vi "MultiChannelFeedbackCooling_aod_feedback(Host).vi"(5 "RIO Device":T1="RIO0") -> ()   [LabVIEW 2014]
doc: "This VI will will initialize the FPGA VI and then continually read and convert single point values from 4 channels of an analog input module."
uses:
  <vilib>/userdefined/High Color/nirio_resource_hc.ctl
  <vilib>/rvi/Analysis/host/Butterworth/config/Butterworth Filter Order.ctl
  <vilib>/rvi/Analysis/host/Butterworth/config/Butterworth Filter Type.ctl
  <vilib>/FPGAPlugInAG/PXI-7854R/niLvFpga_Open_PXI-7854R.vi
  <vilib>/FPGAPlugInAG/PXI-7854R/niLvFpga_Run_PXI-7854R.vi
  <vilib>/rvi/Analysis/host/Butterworth/config/BwScaledCoefficients.vi
  <vilib>/Utility/error.llb/Error Cluster From Error Code.vi
  <vilib>/rvi/errors/niLvFpgaAdjustHostInterfaceError.vi
  <vilib>/Utility/file.llb/Read From Spreadsheet File (I64).vi
  <vilib>/FPGAPlugInAG/PXI-7854R/niLvFpga_Close_PXI-7854R.vi
  <vilib>/rvi/interface/nirviOpenFPGA/nirviOpenFPGA.xnode
  FPGA Bitfiles/MultiChannelFeed_FPGATarget_MultiChannelfFee_WCKCUTTT7ag.lvbitx
  MultiChannelfFeedbackCooling (FPGA).vi
  <vilib>/rvi/interface/nirviMethod/nirviMethod.xnode
  <vilib>/rvi/Analysis/host/Butterworth/XNode/ButterworthCoefficients.xnode
  <vilib>/rvi/interface/nirviReadWriteControl/nirviReadWriteControl.xnode
  <vilib>/rvi/interface/nirviCloseFPGA/nirviCloseFPGA.xnode
  NiFpgaLv.dll
  <vilib>/rvi/Analysis/host/Public/NI_FpgaMspHost.lvlib
panel:
  out "tot_fb_img":i16(graph)
  out "fb_img":i16(graph)
  out "AI_img":i16(graph)=3016
  in  "pg_img":fxp<+/-,24,12>
  in  "dg_img":fxp<+/-,24,12>
  in  "ig_img":fxp<+/-,24,6>
  in  "setpt_img":i16=3000
  in  "Upper lim_img":fxp<+/-,16,16>=1000.0
  in  "Lower lim_img":fxp<+/-,16,16>=-1000.0
  in  "lp freq_img":dbl=5000.0
  in  "hp freq_img":dbl=5000.0
  in  "output offset_img":i16
  in  "End value arb (ch1)":fxp<+/-,32,16>
  in  "Step arb (ch1)":fxp<+/-,32,16>=0.0005035400390625
  in  "Arb gain (ch2)":fxp<+/-,24,12>
  in  "z arb scale":fxp<+/-,33,17>
  in  "ramp arb drive":bool
  in  "End value arb (ch0)":fxp<+/-,32,16>
  in  "Step arb (ch0)":fxp<+/-,32,16>=0.0005035400390625
  in  "Delay Time (s) arb":dbl=0.001 caption="Delay Time (s)"
  in  "Buffer file path":path=path "C:/GitHub/opt_lev/labview/fpga/gauss_cdf.txt"
  in  "Write data to buffers":bool
  in  "Arb steps per cycle":u16=1
  in  "Arb gain (ch1)":fxp<+/-,24,12>
  in  "Arb gain (ch0)":fxp<+/-,24,12>
  in  "power setpt":i16=7000
  in  "Upper lim pow":fxp<+/-,16,16>=10000.0
  in  "Lower lim pow":fxp<+/-,16,16>=-10000.0
  in  "hp freq pow":dbl=5000.0
  in  "lp freq pow":dbl=5000.0
  in  "Use_PID2_power":bool=TRUE
  in  "hp freq 1":dbl=1100.0
  in  "hp freq 0":dbl=1100.0
  in  "lp freq 0":dbl=1100.0
  in  "DC offset 0":i16
  in  "Lower lim 0":fxp<+/-,16,16>=-3600.0
  in  "Upper lim 0":fxp<+/-,16,16>=3600.0
  in  "Dg 0":fxp<+/-,24,12>
  in  "Bead setpt 0":i16
  in  "change pars":bool
  in  "hp freq 2":dbl=1100.0
  in  "lp freq 1":dbl=1100.0
  in  "lp freq 2":dbl=1100.0
  in  "ramp power":bool
  in  "End value power":i16=1600
  in  "Step power":i16=5
  in  "Delay Time (s) power":dbl=0.01 caption="Delay Time (s)"
  in  "Count(usec)":u32=10
  in  "?":u16(ring)=2 items=["Both", "AOD", "Bead"]
  in  "?":u16(ring)=2 items=["Both", "AOD", "Bead"]
  in  "?":u16(ring) items=["Both", "AOD", "Bead"]
  in  "?":u16(ring)=2 items=["Both", "AOD", "Bead"]
  in  "?":u16(ring)=1 items=["Both", "AOD", "Bead"]
  in  "?":u16(ring)=2 items=["Both", "AOD", "Bead"]
  in  "Pg d2":fxp<+/-,24,12>=-6.0
  in  "Ig d2":fxp<+/-,24,6>=-0.7999992370605469
  in  "Dg d2":fxp<+/-,24,12>
  in  "Ig 2":fxp<+/-,24,6>
  in  "DC offset 2":i16=7000
  in  "Lower lim 2":fxp<+/-,16,16>=-2000.0
  in  "Upper lim 2":fxp<+/-,16,16>=2000.0
  in  "Dg 2":fxp<+/-,24,12>
  in  "Pg 2":fxp<+/-,24,12>
  in  "Bead setpt 2":i16=1000
  in  "change pars 2":bool
  in  "change pars 1":bool
  in  "DC offset 1":i16
  in  "Lower lim 1":fxp<+/-,16,16>=-32768.0
  in  "Upper lim 1":fxp<+/-,16,16>=32767.0
  in  "Dg 1":fxp<+/-,24,12>
  in  "Bead setpt 1":i16
  out "Tot feedback + DC, Ch2":i16(graph)=3860
  out "Individual feedback, Ch2":cluster{"fb_0":i16, "fb_d0":i16}(graph)
  out "AI1 2":cluster{"AI2":i16, "AI5":i16}(graph)={"AI2"=2178, "AI5"=2178}
  out "Tot feedback + DC, Ch1":i16(graph)
  out "Individual feedback, Ch1":cluster{"fb_0":i16, "fb_d0":i16}(graph)
  out "AI1":cluster{"AI1":i16, "AI4":i16}(graph)={"AI1"=-1988, "AI4"=-1988}
  out "Tot feedback + DC, Ch0":i16(graph)
  out "Individual feedback, Ch0":cluster{"fb_0":i16, "fb_d0":i16}(graph)
  out "AI0":cluster{"AI0":i16, "AI3":i16}(graph)={"AI0"=-128, "AI3"=-128}
  in  "stop":bool
  # "FPGA feedback GUI"
  # "Bead arbitrary drive:"
  # "PID controls, X (ch 0):"
  # "PID controls, Y (ch 1):"
  # "Bead feedback:"
  # "Bead feedback:"
  # "PID controls, Z (ch 2):"
  # "Bead feedback:"
  # "AOD feeback:"
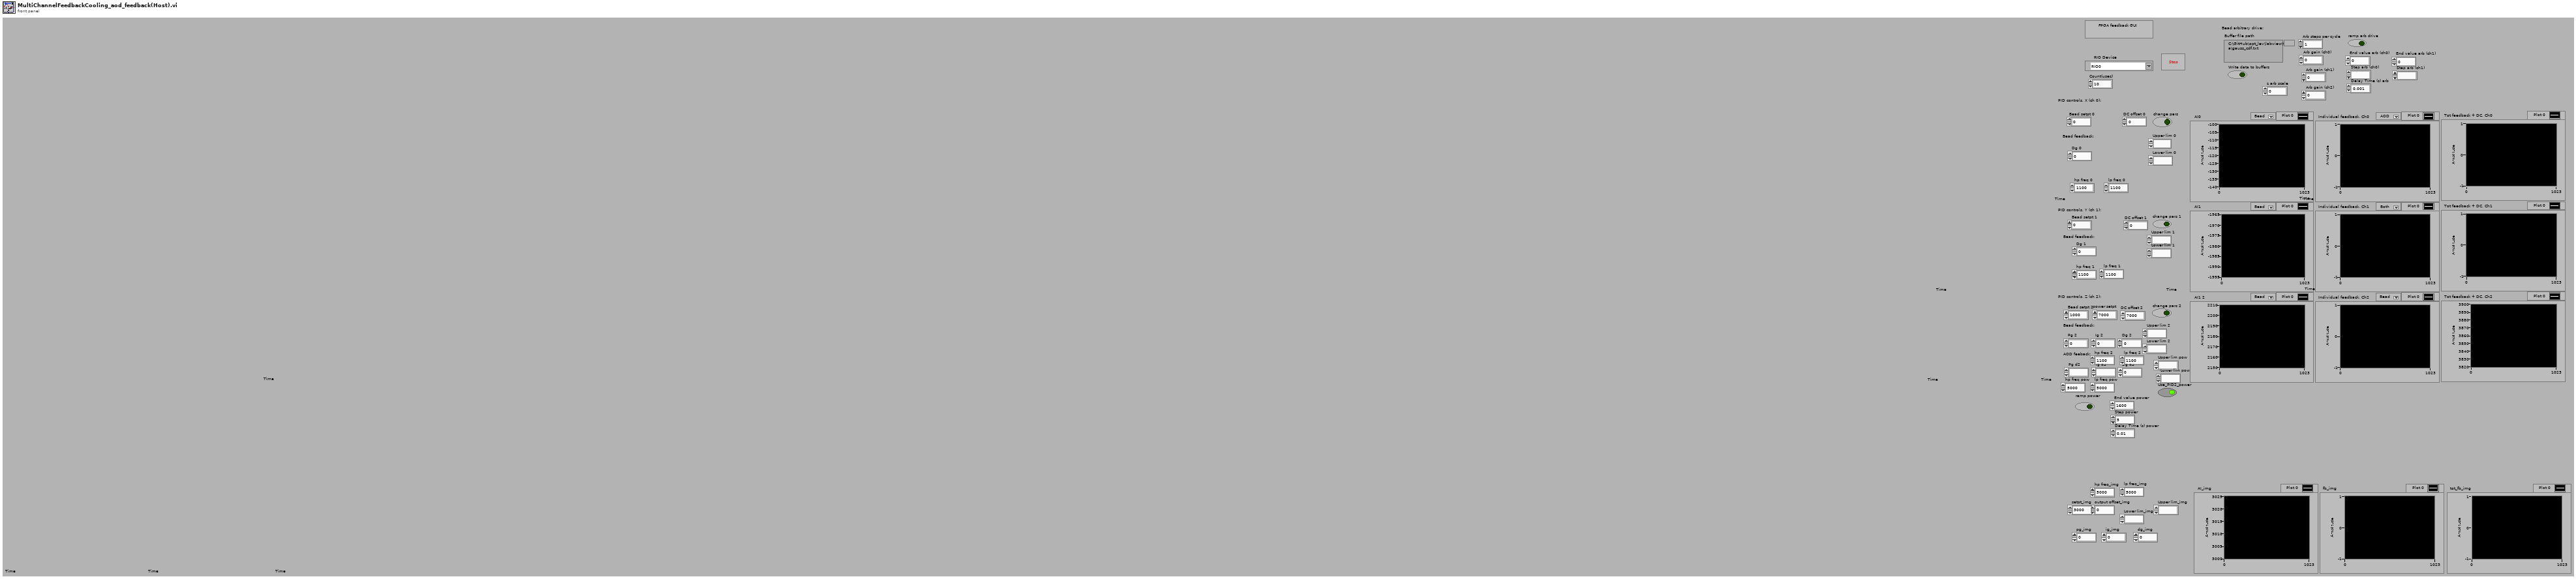
[diagram p1: front panel]
types:
  T1 = typedef "nirio_resource_hc.ctl" = tag
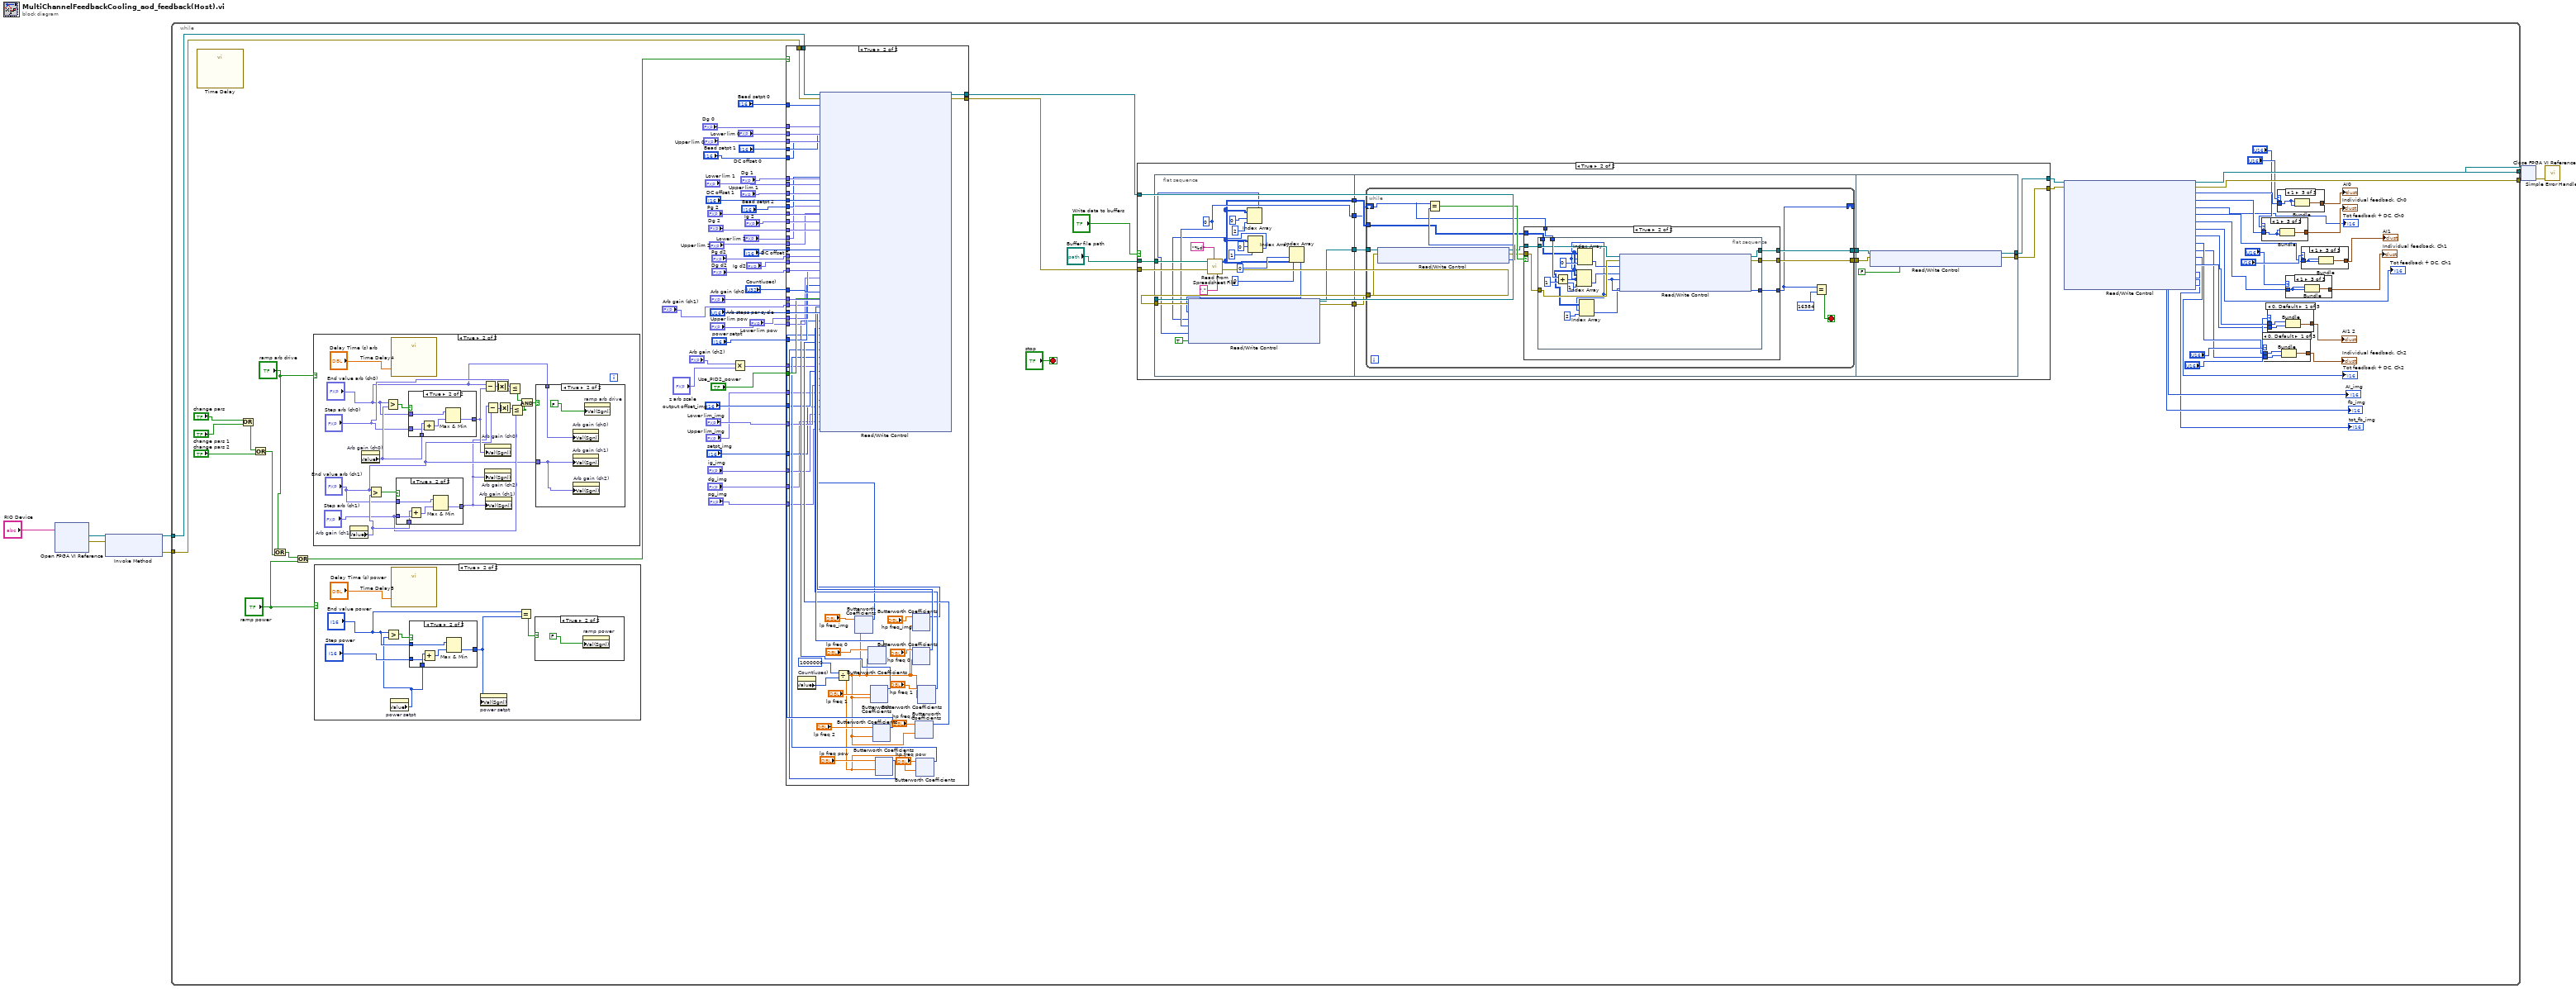
[diagram p0: block diagram]
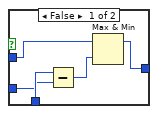
[diagram p4: hidden frame]
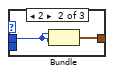
[diagram p5: hidden frame]
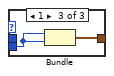
[diagram p6: hidden frame]
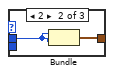
[diagram p7: hidden frame]
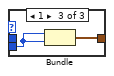
[diagram p8: hidden frame]
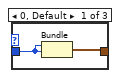
[diagram p9: hidden frame]
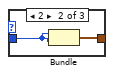
[diagram p10: hidden frame]
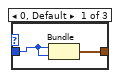
[diagram p11: hidden frame]
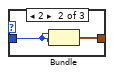
[diagram p12: hidden frame]
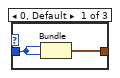
[diagram p13: hidden frame]
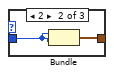
[diagram p14: hidden frame]
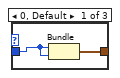
[diagram p15: hidden frame]
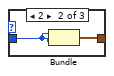
[diagram p16: hidden frame]
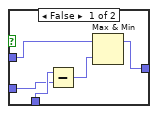
[diagram p18: hidden frame]
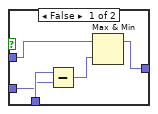
[diagram p20: hidden frame]
diagram:
  n1 = xnode "Open FPGA VI Reference"("resource name"="RIO Device") -> ("FPGA VI Reference Out"=w3:refnum<k20>, "error out"=w2:errorcluster)  [unwired: 1 in]
  n2 = xnode "Invoke Method"("FPGA VI Reference In"=w3, "error in"=w2) -> ("FPGA VI Reference Out"=w5:refnum<k20>, "error out"=w4:errorcluster)  [unwired: 1 in]
  n3 = while {
    tunnel: [w92] -> w8
    tunnel: w5 -> [w84]
    tunnel: w4 -> [w83]
    tunnel: [w91] -> w1
    stop <- "stop" stop-if-true
    n4 = call "Time Delay"() -> ()  [unwired: 11 in, 1 out]
    n5 = Or(x="change pars", y="change pars 1") -> (x .or. y?=w57:bool)
    n6 = Or(x=w57, y="change pars 2") -> (x .or. y?=w23:bool)
    n7 = Or(x="ramp arb drive", y=w23) -> (x .or. y?=w30:bool)
    n8 = Or(x=w30, y="ramp power") -> (x .or. y?=w31:bool)
    n9 = case shown="True" "ramp arb drive" {
      frame False {
      }
      frame True {
        n10 = property on="Arb gain (ch1)" class="DigNum (strict)"() -> ("Value"=w162:fxp<+/-,24,12>)  [unwired: 2 in, 2 out]
        n11 = property on="Arb gain (ch0)" class="DigNum (strict)"() -> ("Value"=w165:fxp<+/-,24,12>)  [unwired: 2 in, 2 out]
        n12 = Greater?(x="End value arb (ch1)", y=w162) -> (0:w163:bool)
        n13 = Greater?(x="End value arb (ch0)", y=w165) -> (0:w166:bool)
        n14 = call "Time Delay4"("Delay Time (s)"="Delay Time (s) arb") -> ()  [unwired: 10 in, 1 out]
        n15 = case shown="True" w163 {
          tunnel: "End value arb (ch1)" -> [w168 w174]
          tunnel: w162 -> [w171 w172]
          tunnel: "Step arb (ch1)" -> [w170 w176]
          tunnel: [w167 w173] -> w149
          frame False {
            n16 = Subtract(x=w171, y=w170) -> (x-y=w169:fxp<+/-,33,17>)
            n17 = Max & Min(x=w168, y=w169) -> (max(x,y)=w167:fxp<+/-,33,17>)  [unwired: 1 out]
          }
          frame True {
            n18 = Add(x=w172, y=w176) -> (x+y=w175:fxp<+/-,33,17>)
            n19 = Max & Min(x=w174, y=w175) -> (min(x,y)=w173:fxp<+/-,33,17>)  [unwired: 1 out]
          }
        }
        n20 = case shown="True" w166 {
          tunnel: "End value arb (ch0)" -> [w181 w186]
          tunnel: w165 -> [w184 w189]
          tunnel: "Step arb (ch0)" -> [w183 w188]
          tunnel: [w180 w185] -> w161
          frame False {
            n21 = Subtract(x=w184, y=w183) -> (x-y=w182:fxp<+/-,33,17>)
            n22 = Max & Min(x=w181, y=w182) -> (max(x,y)=w180:fxp<+/-,33,17>)  [unwired: 1 out]
          }
          frame True {
            n23 = Add(x=w189, y=w188) -> (x+y=w187:fxp<+/-,33,17>)
            n24 = Max & Min(x=w186, y=w187) -> (min(x,y)=w185:fxp<+/-,33,17>)  [unwired: 1 out]
          }
        }
        n25 = Subtract(x="End value arb (ch0)", y=w161) -> (x-y=w160:fxp<+/-,34,18>)
        n26 = property on="Arb gain (ch0)" class="DigNum (strict)"("Val(Sgnl)"=w161) -> ()  [unwired: 2 in, 2 out]
        n27 = property on="Arb gain (ch2)" class="DigNum (strict)"("Val(Sgnl)"=w149) -> ()  [unwired: 2 in, 2 out]
        n28 = Subtract(x=w149, y="End value arb (ch1)") -> (x-y=w157:fxp<+/-,34,18>)
        n29 = property on="Arb gain (ch1)" class="DigNum (strict)"("Val(Sgnl)"=w149) -> ()  [unwired: 2 in, 2 out]
        n30 = Absolute Value(x=w160) -> (abs(x)=w159:fxp<+,33,17>)
        n31 = Absolute Value(x=w157) -> (abs(x)=w156:fxp<+,33,17>)
        n32 = Less Or Equal?(x=w159, y="Step arb (ch0)") -> (x <= y?=w153:bool)
        n33 = Less Or Equal?(x=w156, y="Step arb (ch1)") -> (x <= y?=w152:bool)
        n34 = And(x=w153, y=w152) -> (x .and. y?=w154:bool)
        n35 = case shown="True" w154 {
          tunnel: "End value arb (ch0)" -> [_ w178]
          tunnel: "End value arb (ch1)" -> [_ w177]
          frame False {
          }
          frame True {
            n36 = property on="Arb gain (ch0)" class="DigNum (strict)"("Val(Sgnl)"=w178) -> ()  [unwired: 2 in, 2 out]
            n37 = property on="Arb gain (ch1)" class="DigNum (strict)"("Val(Sgnl)"=w177) -> ()  [unwired: 2 in, 2 out]
            n38 = property on="Arb gain (ch2)" class="DigNum (strict)"("Val(Sgnl)"=w177) -> ()  [unwired: 2 in, 2 out]
            n39 = property on="ramp arb drive" class="Bool (strict)"("Val(Sgnl)"=FALSE) -> ()  [unwired: 2 in, 2 out]
          }
        }
      }
    }
    n40 = case shown="True" "ramp power" {
      frame False {
      }
      frame True {
        n41 = property on="power setpt" class="DigNum (strict)"() -> ("Value"=w94:i16)  [unwired: 2 in, 2 out]
        n42 = Greater?(x="End value power", y=w94) -> (0:w99:bool)
        n43 = call "Time Delay5"("Delay Time (s)"="Delay Time (s) power") -> ()  [unwired: 10 in, 1 out]
        n44 = case shown="True" w99 {
          tunnel: "End value power" -> [w102 w107]
          tunnel: w94 -> [w105 w110]
          tunnel: "Step power" -> [w104 w109]
          tunnel: [w101 w106] -> w93
          frame False {
            n45 = Subtract(x=w105, y=w104) -> (x-y=w103:i16)
            n46 = Max & Min(x=w102, y=w103) -> (max(x,y)=w101:i16)  [unwired: 1 out]
          }
          frame True {
            n47 = Add(x=w110, y=w109) -> (x+y=w108:i16)
            n48 = Max & Min(x=w107, y=w108) -> (min(x,y)=w106:i16)  [unwired: 1 out]
          }
        }
        n49 = property on="power setpt" class="DigNum (strict)"("Val(Sgnl)"=w93) -> ()  [unwired: 2 in, 2 out]
        n50 = Equal?(x="End value power", y=w93) -> (x = y?=w98:bool)
        n51 = case shown="True" w98 {
          frame False {
          }
          frame True {
            n52 = property on="ramp power" class="Bool (strict)"("Val(Sgnl)"=FALSE) -> ()  [unwired: 2 in, 2 out]
          }
        }
      }
    }
    n53 = Multiply(x="Arb gain (ch2)", y="z arb scale") -> (x*y=w20:fxp<+/-,56,28>)
    n54 = case shown="True" w31 {
      tunnel: w83 -> [w271 w326]
      tunnel: [w271 w334] -> w79
      tunnel: [w270 w333] -> w80
      tunnel: "Bead setpt 0" -> [_ w332]
      tunnel: "Dg 0" -> [_ w331]
      tunnel: "Upper lim 0" -> [_ w329]
      tunnel: "Lower lim 0" -> [_ w330]
      tunnel: "DC offset 0" -> [_ w328]
      tunnel: w84 -> [w270 w327]
      tunnel: "Bead setpt 1" -> [_ w325]
      tunnel: "Dg 1" -> [_ w324]
      tunnel: "Lower lim 1" -> [_ w323]
      tunnel: "Upper lim 1" -> [_ w322]
      tunnel: "DC offset 1" -> [_ w321]
      tunnel: "Bead setpt 2" -> [_ w320]
      tunnel: "Pg 2" -> [_ w319]
      tunnel: "Ig 2" -> [_ w318]
      tunnel: "Dg 2" -> [_ w317]
      tunnel: "Lower lim 2" -> [_ w316]
      tunnel: "Upper lim 2" -> [_ w315]
      tunnel: "DC offset 2" -> [_ w314]
      tunnel: "Pg d2" -> [_ w313]
      tunnel: "Ig d2" -> [_ w312]
      tunnel: "Dg d2" -> [_ w311]
      tunnel: "Arb gain (ch0)" -> [_ w310]
      tunnel: "Arb gain (ch1)" -> [_ w296]
      tunnel: "Arb steps per cycle" -> [_ w309]
      tunnel: "Count(usec)" -> [_ w308]
      tunnel: "Use_PID2_power" -> [_ w299]
      tunnel: "Lower lim pow" -> [_ w295]
      tunnel: "Upper lim pow" -> [_ w294]
      tunnel: "power setpt" -> [_ w293]
      tunnel: w20 -> [_ w284]
      tunnel: "output offset_img" -> [_ w283]
      tunnel: "Lower lim_img" -> [_ w278]
      tunnel: "Upper lim_img" -> [_ w277]
      tunnel: "setpt_img" -> [_ w275]
      tunnel: "ig_img" -> [_ w274]
      tunnel: "dg_img" -> [_ w273]
      tunnel: "pg_img" -> [_ w272]
      frame False {
      }
      frame True {
        n55 = property on="Count(usec)" class="DigNum (strict)"() -> ("Value"=w304:u32)  [unwired: 2 in, 2 out]
        n56 = Divide(x=u32 1000000, y=w304) -> (x/y=w281:dbl)
        n57 = xnode "Butterworth Coefficients"("cutoff frequency (Hz)"="lp freq_img", "sample rate (S/s)"=w281) -> ("scaled coefficients"=w276:i32[])  [unwired: 1 in, 1 out]
        n58 = xnode "Butterworth Coefficients"("cutoff frequency (Hz)"="lp freq 0", "sample rate (S/s)"=w281) -> ("scaled coefficients"=w292:i32[])  [unwired: 1 in, 1 out]
        n59 = xnode "Butterworth Coefficients"("cutoff frequency (Hz)"="lp freq 1", "sample rate (S/s)"=w281) -> ("scaled coefficients"=w290:i32[])  [unwired: 1 in, 1 out]
        n60 = xnode "Butterworth Coefficients"("cutoff frequency (Hz)"="lp freq 2", "sample rate (S/s)"=w281) -> ("scaled coefficients"=w288:i32[])  [unwired: 1 in, 1 out]
        n61 = xnode "Butterworth Coefficients"("cutoff frequency (Hz)"="lp freq pow", "sample rate (S/s)"=w281) -> ("scaled coefficients"=w286:i32[])  [unwired: 1 in, 1 out]
        n62 = xnode "Butterworth Coefficients"("cutoff frequency (Hz)"="hp freq_img", "sample rate (S/s)"=w281) -> ("scaled coefficients"=w279:i32[])  [unwired: 1 in, 1 out]
        n63 = xnode "Butterworth Coefficients"("cutoff frequency (Hz)"="hp freq 0", "sample rate (S/s)"=w281) -> ("scaled coefficients"=w291:i32[])  [unwired: 1 in, 1 out]
        n64 = xnode "Butterworth Coefficients"("cutoff frequency (Hz)"="hp freq 2", "sample rate (S/s)"=w281) -> ("scaled coefficients"=w287:i32[])  [unwired: 1 in, 1 out]
        n65 = xnode "Butterworth Coefficients"("cutoff frequency (Hz)"="hp freq pow", "sample rate (S/s)"=w281) -> ("scaled coefficients"=w285:i32[])  [unwired: 1 in, 1 out]
        n66 = xnode "Butterworth Coefficients"("cutoff frequency (Hz)"="hp freq 1", "sample rate (S/s)"=w281) -> ("scaled coefficients"=w289:i32[])  [unwired: 1 in, 1 out]
        n67 = xnode "Read/Write Control"("FPGA VI Reference In"=w327, "error in"=w326, "Dc Pos 0"=w332, "dg 0"=w331, "Lower lim 0"=w330, "Upper lim 0"=w329, "output offset 0"=w328, "Dc Pos 1"=w325, "dg 1"=w324, "Lower lim 1"=w323, "Upper lim 1"=w322, "output offset 1"=w321, "Dc Pos 2"=w320, "pg 2"=w319, "ig 3"=w318, "dg 2"=w317, "Lower lim 2"=w316, "Upper lim 2"=w315, "output offset 2"=w314, "pg d0 3"=w313, "ig d03"=w312, "dg d0 3"=w311, "Arb gain (ch0)"=w310, "Arb gain (ch1)"=w296, "Arb steps per cycle"=w309, "Lower lim 4"=w295, "Upper lim d0 3"=w294, "Dc Pos d2"=w293, "Count(uSec)"=w308, "Use_PID2_X 2"=w299, "lp coeff 0"=w292, "hp coeff 0"=w291, "lp coeff 1"=w290, "hp coeff 1"=w289, "lp coeff 2"=w288, "hp coeff 2"=w287, "lp coeff d2"=w286, "hp coeff d2"=w285, "Arb gain (ch2)"=w284, "output offset_img"=w283, "hp coeff_img"=w279, "Lower lim_img"=w278, "Upper lim_img"=w277, "lp coeff_img"=w276, "setpt_img"=w275, "ig_img"=w274, "dg_img"=w273, "pg_img"=w272) -> ("FPGA VI Reference Out"=w333:refnum<k20>, "error out"=w334:errorcluster)
      }
    }
    n68 = case shown="True" "Write data to buffers" {
      tunnel: "Buffer file path" -> [_ w202]
      tunnel: w80 -> [w191 w201]
      tunnel: w79 -> [w190 w200]
      tunnel: [w191 w193] -> w78
      tunnel: [w190 w192] -> w77
      frame False {
      }
      frame True {
        n69 = flat-sequence {
          tunnel: w202 -> [w221]
          tunnel: w201 -> [w219]
          tunnel: w200 -> [w218]
          tunnel: [w213] -> w199
          tunnel: [w212] -> w198
          tunnel: [w206] -> w197
          tunnel: [w211] -> w196
          tunnel: w199 -> [w227]
          tunnel: w198 -> [w226]
          tunnel: w197 -> [w225]
          tunnel: w196 -> [w224]
          tunnel: [w223] -> w195
          tunnel: [w222] -> w194
          tunnel: w195 -> [w269]
          tunnel: w194 -> [w268]
          tunnel: [w267] -> w193
          tunnel: [w266] -> w192
          frame #0 {
            w211 = 0
            n70 = call-poly <vilib>:"Read From Spreadsheet File.vi"("delimiter (\\t)"="," ("delimiter (\\t)"), "format (%d)"="%d", "file path (dialog if empty)"=w221) -> ("all rows"=w206:i64[][])  [unwired: 4 in, 4 out]
            n71 = Index Array(array=w206, index (row)=0, index (col)=2 ("disabled index (col)")) -> (element=w203:i64)
            n72 = Index Array(array=w206, index (row)=0, index (col)=1 ("disabled index (col)")) -> (element=w209:i64)
            n73 = Index Array(array=w206, index (row)=0, index (col)=0 ("disabled index (col)")) -> (element=w210:i64)
            n74 = xnode "Read/Write Control"("FPGA VI Reference In"=w219, "error in"=w218, "data_buffer_1"=w210, "data_buffer2"=w209, "write_address"=w211, "data_buffer3"=w203, "ready_to_write"=TRUE) -> ("FPGA VI Reference Out"=w212:refnum<k20>, "error out"=w213:errorcluster)
          }
          frame #1 {
            n75 = while {
              shift-right: [w228] -> _
              shift-left: w224 -> [w236]
              tunnel: w226 -> [w240]
              tunnel: w227 -> [w239]
              tunnel: w225 -> [w235]
              tunnel: [w230] -> w223
              tunnel: [w229] -> w222
              stop <- w231 stop-if-true
              n76 = xnode "Read/Write Control"("FPGA VI Reference In"=w240, "error in"=w239) -> ("FPGA VI Reference Out"=w234:refnum<k20>, "error out"=w233:errorcluster, "written_address"=w238:u32)
              n77 = Equal?(x=w236, y=w238) -> (x = y?=w237:bool)
              n78 = case shown="True" w237 {
                tunnel: w236 -> [w243 w250]
                tunnel: w235 -> [_ w249]
                tunnel: w234 -> [w242 w248]
                tunnel: w233 -> [w241 w247]
                tunnel: [w243 w246] -> w228
                tunnel: [w242 w245] -> w230
                tunnel: [w241 w244] -> w229
                frame False {
                }
                frame True {
                  n79 = flat-sequence {
                    tunnel: w250 -> [w263]
                    tunnel: w249 -> [w253]
                    tunnel: w248 -> [w260]
                    tunnel: w247 -> [w259]
                    tunnel: [w252] -> w246
                    tunnel: [w257] -> w245
                    tunnel: [w256] -> w244
                    frame #0 {
                      n80 = Add(x=w263, y=1) -> (x+y=w252:i32)
                      n81 = Index Array(array=w253, index (row)=w252, index (col)=1 ("disabled index (col)")) -> (element=w258:i64)
                      n82 = Index Array(array=w253, index (row)=w252, index (col)=0 ("disabled index (col)")) -> (element=w255:i64)
                      n83 = Index Array(array=w253, index (row)=w252, index (col)=2) -> (element=w251:i64)
                      n84 = xnode "Read/Write Control"("FPGA VI Reference In"=w260, "error in"=w259, "data_buffer_1"=w255, "data_buffer2"=w258, "write_address"=w252, "data_buffer3"=w251) -> ("FPGA VI Reference Out"=w257:refnum<k20>, "error out"=w256:errorcluster)
                    }
                  }
                }
              }
              n85 = Equal?(x=w228, y=u16 16384) -> (x = y?=w231:bool)
            }
          }
          frame #2 {
            n86 = xnode "Read/Write Control"("FPGA VI Reference In"=w269, "error in"=w268, "ready_to_write"=FALSE) -> ("FPGA VI Reference Out"=w267:refnum<k20>, "error out"=w266:errorcluster)
          }
        }
      }
    }
    n87 = xnode "Read/Write Control"("FPGA VI Reference In"=w78, "error in"=w77) -> ("FPGA VI Reference Out"=w92:refnum<k20>, "error out"=w91:errorcluster, "AI0"=w54:i16, "fb_0"=w49:i16, "tot_fb_0"=→"Tot feedback + DC, Ch0":i16, "AI1"=w46:i16, "fb_1"=w44:i16, "tot_fb_1"=→"Tot feedback + DC, Ch1":i16, "AI2"=w41:i16, "fb_2"=w37:i16, "fb_d2"=w36:i16, "tot_fb_2"=→"Tot feedback + DC, Ch2":i16, "AI5"=w38:i16, "AI_img"=→"AI_img":i16, "fb_img"=→"fb_img":i16, "tot_fb_img"=→"tot_fb_img":i16)
    n88 = case shown="1" "?" {
      tunnel: w49 -> [w138 w139 w142]
      tunnel: [w137 w140 w141] -> w51
      frame 0, Default {
        n89 = Bundle("fb_0"=w138, "fb_0"=w138) -> (w137:cluster{"fb_0":i16, "fb_0":i16})  [unwired: 1 in]
      }
      frame 2 {
        n90 = Bundle("fb_0"=w139, "fb_0"=w139) -> (w140:cluster{"fb_0":i16, "fb_0":i16})  [unwired: 1 in]
      }
      frame 1 {
        n91 = Bundle("fb_0"=w142, "fb_0"=w142) -> (w141:cluster{"fb_0":i16, "fb_0":i16})  [unwired: 1 in]
      }
    }
    "Individual feedback, Ch0" <- w51
    n92 = case shown="0, Default" "?" {
      tunnel: w37 -> [w113 w114 _]
      tunnel: w36 -> [w112 _ w117]
      tunnel: [w111 w115 w116] -> w34
      frame 0, Default {
        n93 = Bundle("fb_2"=w113, "fb_d2"=w112) -> (w111:cluster{"fb_2":i16, "fb_d2":i16})  [unwired: 1 in]
      }
      frame 2 {
        n94 = Bundle("fb_2"=w114, "fb_2"=w114) -> (w115:cluster{"fb_2":i16, "fb_2":i16})  [unwired: 1 in]
      }
      frame 1 {
        n95 = Bundle("fb_d2"=w117, "fb_d2"=w117) -> (w116:cluster{"fb_d2":i16, "fb_d2":i16})  [unwired: 1 in]
      }
    }
    "Individual feedback, Ch2" <- w34
    n96 = case shown="0, Default" "?" {
      tunnel: w41 -> [w120 w121 _]
      tunnel: w38 -> [w119 _ w124]
      tunnel: [w118 w122 w123] -> w33
      frame 0, Default {
        n97 = Bundle("AI2"=w120, "AI5"=w119) -> (w118:cluster{"AI2":i16, "AI5":i16})  [unwired: 1 in]
      }
      frame 2 {
        n98 = Bundle("AI2"=w121, "AI2"=w121) -> (w122:cluster{"AI2":i16, "AI2":i16})  [unwired: 1 in]
      }
      frame 1 {
        n99 = Bundle("AI5"=w124, "AI5"=w124) -> (w123:cluster{"AI5":i16, "AI5":i16})  [unwired: 1 in]
      }
    }
    "AI1 2" <- w33
    n100 = case shown="1" "?" {
      tunnel: w54 -> [w144 w145 w148]
      tunnel: [w143 w146 w147] -> w53
      frame 0, Default {
        n101 = Bundle("AI0"=w144, "AI0"=w144) -> (w143:cluster{"AI0":i16, "AI0":i16})  [unwired: 1 in]
      }
      frame 2 {
        n102 = Bundle("AI0"=w145, "AI0"=w145) -> (w146:cluster{"AI0":i16, "AI0":i16})  [unwired: 1 in]
      }
      frame 1 {
        n103 = Bundle("AI0"=w148, "AI0"=w148) -> (w147:cluster{"AI0":i16, "AI0":i16})  [unwired: 1 in]
      }
    }
    "AI0" <- w53
    n104 = case shown="1" "?" {
      tunnel: w44 -> [w125 w127 w130]
      tunnel: [w126 w128 w129] -> w43
      frame 0, Default {
        n105 = Bundle("fb_1"=w125, "fb_1"=w125) -> (w126:cluster{"fb_1":i16, "fb_1":i16})  [unwired: 1 in]
      }
      frame 2 {
        n106 = Bundle("fb_1"=w127, "fb_1"=w127) -> (w128:cluster{"fb_1":i16, "fb_1":i16})  [unwired: 1 in]
      }
      frame 1 {
        n107 = Bundle("fb_1"=w130, "fb_1"=w130) -> (w129:cluster{"fb_1":i16, "fb_1":i16})  [unwired: 1 in]
      }
    }
    "Individual feedback, Ch1" <- w43
    n108 = case shown="1" "?" {
      tunnel: w46 -> [w131 w133 w135]
      tunnel: [w132 w134 w136] -> w32
      frame 0, Default {
        n109 = Bundle("AI1"=w131, "AI1"=w131) -> (w132:cluster{"AI1":i16, "AI1":i16})  [unwired: 1 in]
      }
      frame 2 {
        n110 = Bundle("AI1"=w133, "AI1"=w133) -> (w134:cluster{"AI1":i16, "AI1":i16})  [unwired: 1 in]
      }
      frame 1 {
        n111 = Bundle("AI1"=w135, "AI1"=w135) -> (w136:cluster{"AI1":i16, "AI1":i16})  [unwired: 1 in]
      }
    }
    "AI1" <- w32
  }
  n112 = xnode "Close FPGA VI Reference"("FPGA VI Reference In"=w8, "error in"=w1) -> ("error out"=w7:errorcluster)
  n113 = call <vilib>:"Simple Error Handler.vi"("error in (no error)"=w7) -> ()  [unwired: 4 in, 5 out]
